vi "Debug.vi"   [LabVIEW 2012]
uses:
  <vilib>/Rock Robotics/WPI/Solenoid/WPI_SolenoidValue.ctl
  <vilib>/Rock Robotics/WPI/Relay/WPI_RelayValue.ctl
  Robot Global Data.vi
  <vilib>/Rock Robotics/WPI/Solenoid/WPI_SolenoidSetEnum.vi
  <vilib>/Rock Robotics/WPI/Joystick/WPI_JoystickGetSetRefNum.vi
  <vilib>/Rock Robotics/WPI/RobotDrive/WPI_RobotDriveGetSetRefNum.vi
types:
  T1 = typedef "WPI_JoystickDevRef.ctl" = cluster{"Device":T2}
  T2 = typedef "WPI_JoystickDeviceEnum.ctl" = enum16{"USB 1", "USB 2", "USB 3", "USB 4", "Kinect 1", "Kinect 2"}
  T3 = typedef "WPI_JoystickButtonState.ctl" = cluster{"Button 1":bool, "Button 2":bool, "Button 3":bool, "Button 4":bool, "Button 5":bool, "Button 6":bool, "Button 7":bool, "Button 8":bool, "Button 9":bool, "Button 10":bool, "Button 11":bool, "Button 12":bool}
  T4 = cluster{"axis 1 (x)":dbl, "axis 2 (y)":dbl, "axis 3 (throttle)":dbl, "axis 4":dbl, "axis 5":dbl, "axis 6":dbl}
  T5 = typedef "WPI_RobotDriveDevRef.ctl" = cluster{"DevStatus":errorcluster, "Motors[]":T6[], "Square Inputs":bool, "Max Output":dbl, "Isochronous":bool}
  T6 = typedef "WPI_MotorControlDeviceRef.ctl" = cluster{"DeviceStatus":errorcluster, "Type":enum16{"PWM", "CAN"}, "PWM":cluster{"Digital Module":T7, "PWM Channel":T8, "DeadBand":T9}, "CAN":cluster{"Device Number":u8, "Control Mode":T10, "Semaphore":T11, "Max Vout":dbl}, "Invert":bool, "TransformRef":T12, "InvTransformRef":T12}
  T7 = typedef "FPGA_TypedefDigitalModule.ctl" = enum16{"Digital Module 1", "Digital Module 2"}
  T8 = typedef "FPGA_DIOPWMChannel.ctl" = enum8{"PWM 1", "PWM 2", "PWM 3", "PWM 4", "PWM 5", "PWM 6", "PWM 7", "PWM 8", "PWM 9", "PWM 10", "Invalid"}
  T9 = typedef "WPI_PWMDeadband.ctl" = cluster{"Name":string, "maxPositivePwm":i32, "minPositivePwm":i32, "centerPwm":i32, "maxNegativePwm":i32, "minNegativePwm":i32, "angularRange":u16}
  T10 = typedef "WPI_CANJaguar_ControlMode.ctl" = enum8{"Percent VBus", "Current", "Speed", "Position", "Voltage"}
  T11 = typedef "Semaphore RefNum" = refnum<k1>
  T12 = typedef "WPI_PWMTransform_ConPane.ctl" = refnum<vi>
  T13 = typedef "WPI_SolenoidValue.ctl" = enum16{"Off", "On", "Forward", "Reverse"}
  T14 = typedef "WPI_RelayValue.ctl" = enum16{"Off", "On", "Forward", "Reverse"}
  T15 = typedef "WPI_SolenoidDevRef.ctl" = cluster{"DevStatus":errorcluster, "Solenoid Module":T16, "Forward Solenoid Channel":T17, "Reverse Solenoid Channel":T17}
  T16 = typedef "FPGA_TypedefSolenoidModule.ctl" = enum16{"Solenoid Module 1", "Solenoid Module 2"}
  T17 = typedef "WPI_SolenoidChannel.ctl" = enum8{"Solenoid 1", "Solenoid 2", "Solenoid 3", "Solenoid 4", "Solenoid 5", "Solenoid 6", "Solenoid 7", "Solenoid 8", "Invalid"}
  T18 = typedef "WPI_RelayDevRef.ctl" = cluster{"DevStatus":errorcluster, "Relay Channel":T19, "Digital Module":T7, "Relay Direction":T20}
  T19 = typedef "FPGA_DIORelayChannel.ctl" = enum8{"Relay 1", "Relay 2", "Relay 3", "Relay 4", "Relay 5", "Relay 6", "Relay 7", "Relay 8", "Invalid"}
  T20 = typedef "WPI_RelayDirection.ctl" = enum16{"Both directions", "Forward only", "Reverse only"}
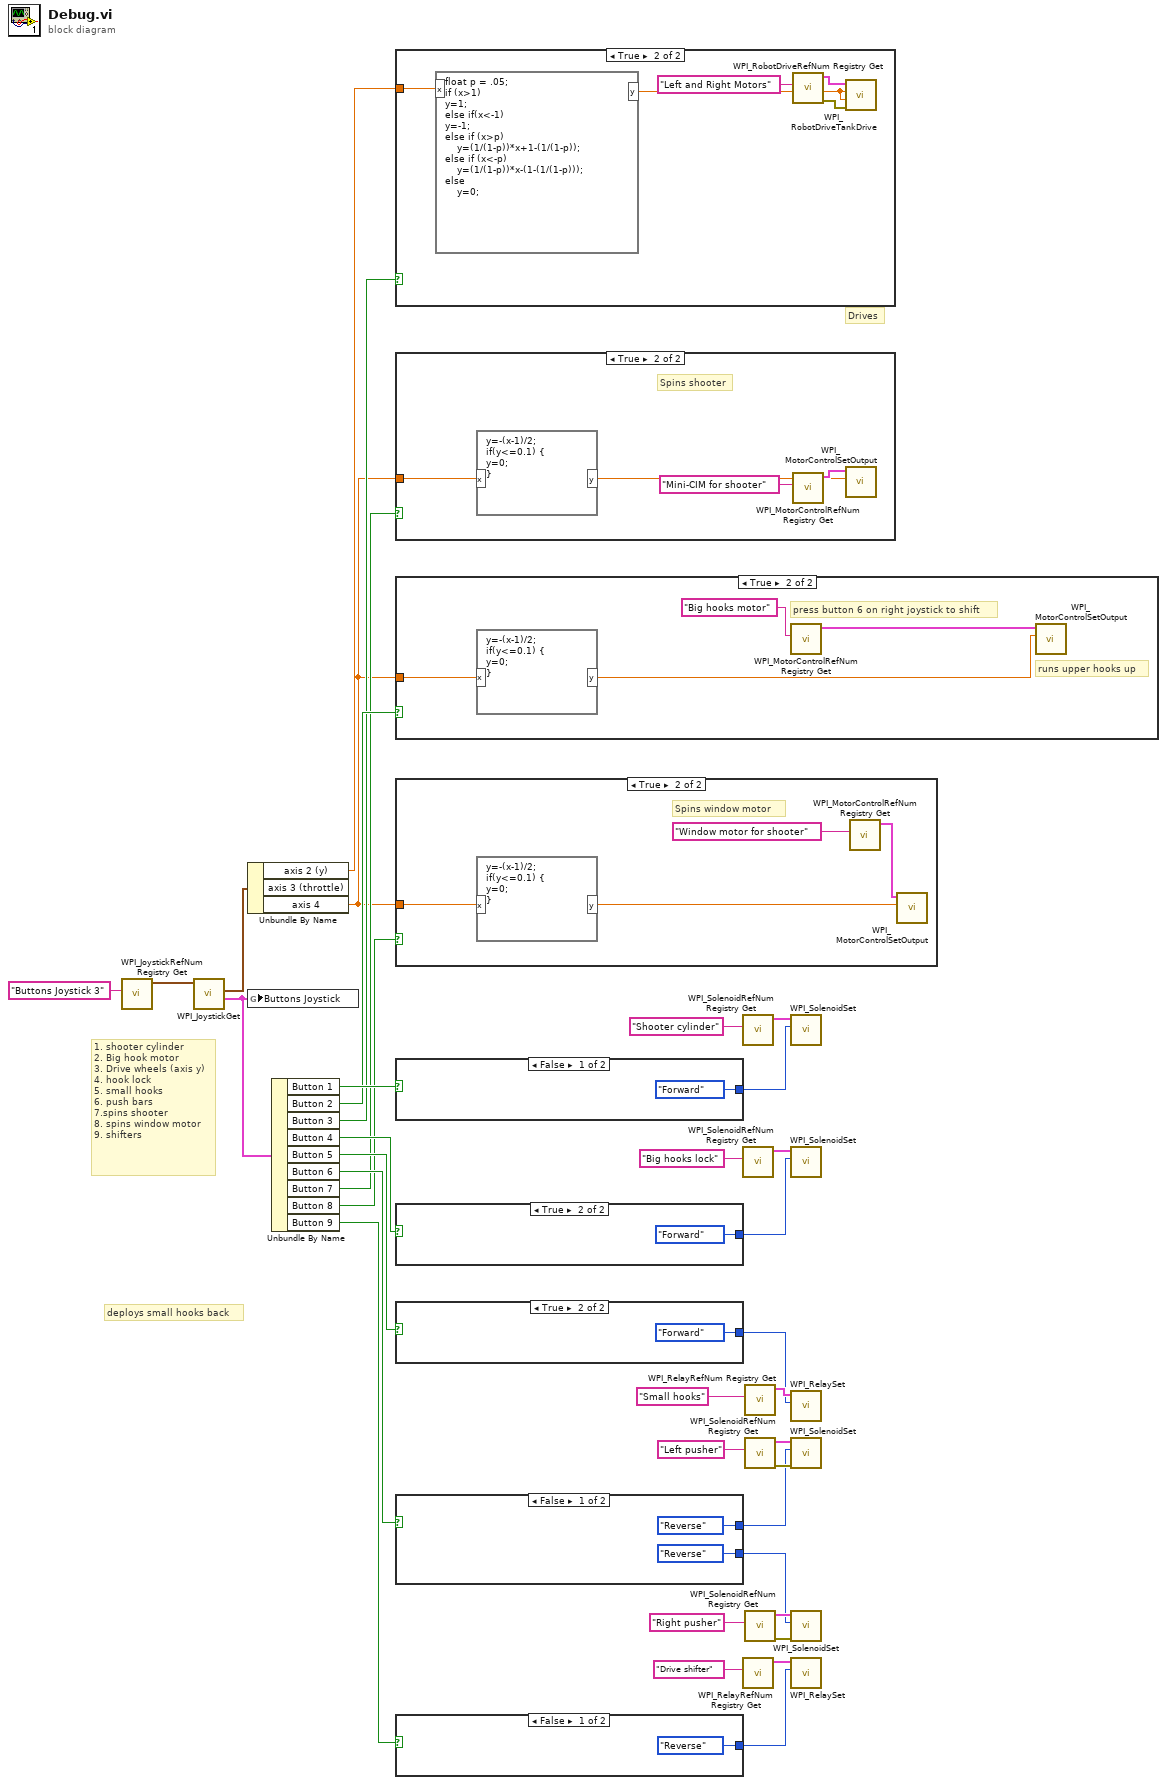
[diagram p0: block diagram]
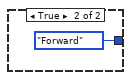
[diagram p2: hidden frame]
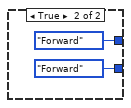
[diagram p5: hidden frame]
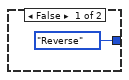
[diagram p6: hidden frame]
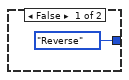
[diagram p7: hidden frame]
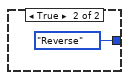
[diagram p10: hidden frame]
diagram:
  # "deploys small hooks back"
  # "1. shooter cylinder\n2. Big hook motor\n3. Drive wheels (axis y)\n4. hook lock\n5. small hooks\n6. push bars\n7.spins shooter\n8. spins window motor\n9. shifters"
  # "Drives"
  n1 = call <vilib>:"WPI_JoystickRefNum Registry Get.vi"("refnum name"="Buttons Joystick 3") -> ("JoystickDevRef"=w35:T1)  [unwired: 1 in, 9 out]
  n2 = call <vilib>:"WPI_JoystickGet.vi"("JoystickDevRef"=w35) -> ("Buttons"=w32:T3, "Axes"=w33:T4)  [unwired: 1 in, 4 out]
  n3 = Unbundle By Name(w33) -> ("axis 2 (y)"=w28:dbl, "axis 4"=w21:dbl)  [unwired: 1 out]
  n4 = global write "Robot Global Data.vi" "Buttons Joystick"(w32) -> ()
  n5 = Unbundle By Name(w32) -> ("Button 1"=w31:bool, "Button 2"=w30:bool, "Button 3"=w29:bool, "Button 4"=w27:bool, "Button 5"=w26:bool, "Button 6"=w25:bool, "Button 7"=w24:bool, "Button 8"=w23:bool, "Button 9"=w22:bool)
  n6 = case shown="True" w29 {
    tunnel: w28 -> [_ w37]
    frame False {
    }
    frame True {
      n7 = formula code="float p = .05; \nif (x>1)\ny=1;\nelse if(x<-1)\ny=-1;\nelse if (x>p)\n    y=(1/(1-p))*x+1-(1/(1-p));\nelse if (x<-p) \n    y=(1/(1-p))*x-(1-(1/(1-p)));\nelse\n    y=0;"("x"=w37) -> ("y"=w36:dbl)
      n8 = call <vilib>:"WPI_RobotDriveRefNum Registry Get.vi"("refnum name"="Left and Right Motors") -> ("error out"=w40:errorcluster, "RobotDriveDevRef"=w39:T5)  [unwired: 1 in, 8 out]
      n9 = call <vilib>:"WPI_RobotDriveTankDrive.vi"("error in (no error)"=w40, "Right axis value"=w36, "Left axis value"=w36, "RobotDriveDevRef"=w39) -> ()  [unwired: 5 in, 3 out]
    }
  }
  n10 = case shown="True" w24 {
    tunnel: w21 -> [_ w42]
    frame False {
    }
    frame True {
      # "Spins shooter"
      n11 = formula code="y=-(x-1)/2;\nif(y<=0.1) {\ny=0;\n}"("x"=w42) -> ("y"=w41:dbl)
      n12 = call <vilib>:"WPI_MotorControlRefNum Registry Get.vi"("refnum name"="Mini-CIM for shooter") -> ("MotorControlDevRef"=w43:T6)  [unwired: 9 in, 1 out]
      n13 = call <vilib>:"WPI_MotorControlSetOutput.vi"("Output"=w41, "MotorControlDevRef"=w43) -> ()  [unwired: 7 in, 3 out]
    }
  }
  n14 = case shown="True" w30 {
    tunnel: w21 -> [_ w46]
    frame False {
    }
    frame True {
      # "press button 6 on right joystick to shift"
      # "runs upper hooks up"
      n15 = formula code="y=-(x-1)/2;\nif(y<=0.1) {\ny=0;\n}"("x"=w46) -> ("y"=w45:dbl)
      n16 = call <vilib>:"WPI_MotorControlRefNum Registry Get.vi"("refnum name"="Big hooks motor") -> ("MotorControlDevRef"=w47:T6)  [unwired: 9 in, 1 out]
      n17 = call <vilib>:"WPI_MotorControlSetOutput.vi"("Output"=w45, "MotorControlDevRef"=w47) -> ()  [unwired: 7 in, 3 out]
    }
  }
  n18 = case shown="True" w23 {
    tunnel: w21 -> [_ w50]
    frame False {
    }
    frame True {
      # "Spins window motor"
      n19 = formula code="y=-(x-1)/2;\nif(y<=0.1) {\ny=0;\n}"("x"=w50) -> ("y"=w49:dbl)
      n20 = call <vilib>:"WPI_MotorControlRefNum Registry Get.vi"("refnum name"="Window motor for shooter") -> ("MotorControlDevRef"=w51:T6)  [unwired: 9 in, 1 out]
      n21 = call <vilib>:"WPI_MotorControlSetOutput.vi"("Output"=w49, "MotorControlDevRef"=w51) -> ()  [unwired: 7 in, 3 out]
    }
  }
  n22 = case shown="False" w31 {
    tunnel: [WPI_SolenoidValue."Forward" ("Value") WPI_SolenoidValue."Reverse" ("Value")] -> w19
    frame False {
    }
    frame True {
    }
  }
  n23 = case shown="True" w27 {
    tunnel: [WPI_SolenoidValue."Reverse" ("Value") WPI_SolenoidValue."Forward" ("Value")] -> w15
    frame False {
    }
    frame True {
    }
  }
  n24 = case shown="True" w26 {
    tunnel: [WPI_RelayValue."Reverse" ("RelayValue") WPI_RelayValue."Forward" ("RelayValue")] -> w12
    frame False {
    }
    frame True {
    }
  }
  n25 = case shown="False" w25 {
    tunnel: [WPI_SolenoidValue."Reverse" ("Value") WPI_SolenoidValue."Forward" ("Value")] -> w1
    tunnel: [WPI_SolenoidValue."Reverse" ("Value") WPI_SolenoidValue."Forward" ("Value")] -> w2
    frame False {
    }
    frame True {
    }
  }
  n26 = case shown="False" w22 {
    tunnel: [WPI_RelayValue."Reverse" ("RelayValue") WPI_RelayValue."Forward" ("RelayValue")] -> w9
    frame False {
    }
    frame True {
    }
  }
  n27 = call <vilib>:"WPI_SolenoidRefNum Registry Get.vi"("refnum name"="Shooter cylinder") -> ("SolenoidDevRef"=w18:T15)  [unwired: 9 in, 1 out]
  n28 = call <vilib>:"WPI_SolenoidRefNum Registry Get.vi"("refnum name"="Big hooks lock") -> ("SolenoidDevRef"=w17:T15)  [unwired: 9 in, 1 out]
  n29 = call <vilib>:"WPI_RelayRefNum Registry Get.vi"("refnum name"="Drive shifter") -> ("RelayDevRef"=w10:T18)  [unwired: 9 in, 1 out]
  n30 = call <vilib>:"WPI_RelayRefNum Registry Get.vi"("refnum name"="Small hooks") -> ("RelayDevRef"=w13:T18)  [unwired: 9 in, 1 out]
  n31 = call <vilib>:"WPI_SolenoidRefNum Registry Get.vi"("refnum name"="Left pusher") -> ("error out"=w5:errorcluster, "SolenoidDevRef"=w4:T15)  [unwired: 9 in]
  n32 = call <vilib>:"WPI_SolenoidRefNum Registry Get.vi"("refnum name"="Right pusher") -> ("error out"=w8:errorcluster, "SolenoidDevRef"=w7:T15)  [unwired: 9 in]
  n33 = call-poly <vilib>:"WPI_SolenoidSet.vi"("Value"=w19, "SolenoidDevRef"=w18) -> ()  [unwired: 8 in, 2 out]
  n34 = call-poly <vilib>:"WPI_SolenoidSet.vi"("Value"=w15, "SolenoidDevRef"=w17) -> ()  [unwired: 8 in, 2 out]
  n35 = call <vilib>:"WPI_RelaySet.vi"("RelayValue"=w12, "RelayDevRef"=w13) -> ()  [unwired: 8 in, 2 out]
  n36 = call-poly <vilib>:"WPI_SolenoidSet.vi"("error in (no error)"=w5, "Value"=w1, "SolenoidDevRef"=w4) -> ()  [unwired: 7 in, 2 out]
  n37 = call-poly <vilib>:"WPI_SolenoidSet.vi"("error in (no error)"=w8, "Value"=w2, "SolenoidDevRef"=w7) -> ()  [unwired: 7 in, 2 out]
  n38 = call <vilib>:"WPI_RelaySet.vi"("RelayValue"=w9, "RelayDevRef"=w10) -> ()  [unwired: 8 in, 2 out]
